vi "PointsToTiming.vi"(6 "Timing":T1 {"Pre-trigger length" format="%#_4p"; "Record length" format="%#_6p"; "Data rate" format="%#_6p"}, 7 "Device":T2, 8 "Pre-trigger position, %":dbl=1000000.0, 9 "Pre-trigger points":i64, 10 "Total points":i64, 11 "Actual Rate, Hz":dbl) -> (0 "Timing out":T1 {"Pre-trigger length" format="%#_4p"; "Record length" format="%#_6p"; "Data rate" format="%#_6p"}, 1 "Pre-trigger length, s":dbl, 2 "Record length, s":dbl, 3 "Data rate, Hz":dbl)   [LabVIEW 2015]
uses:
  Utilities/Controls/Timing Element.ctl
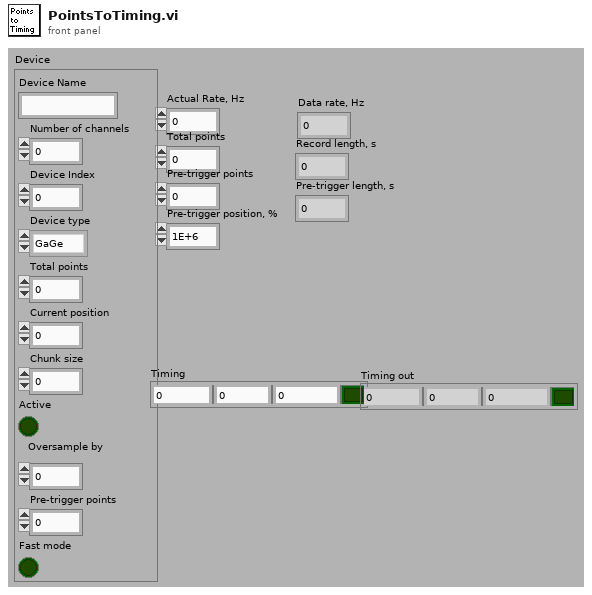
[diagram p1: front panel]
types:
  T1 = typedef "Timing Element.ctl" = cluster{"Data rate":dbl, "Record length":dbl, "Pre-trigger length":dbl, "Ext. clock":bool}
  T2 = cluster{"Device Name":string, "Number of channels":i32, "Device Index":i32, "Device type":enum16{"GaGe", "NI-DAQ", "NI-Scope", "CAMAC", "VXI-1433", "VXI-1437"}, "Total points":i64, "Current position":i64, "Chunk size":i64, "Active":bool, "Oversample by":i32, "Pre-trigger points":i64, "Fast mode":bool}
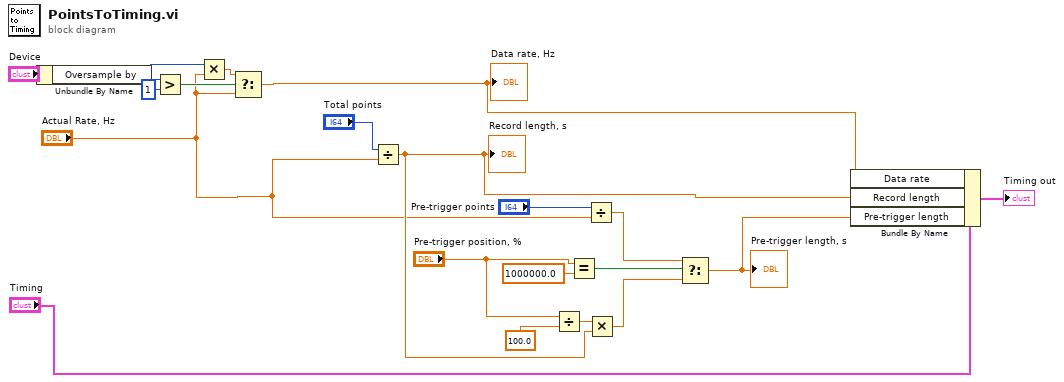
[diagram p0: block diagram]
diagram:
  n1 = Unbundle By Name("Device") -> ("Oversample by"=w2:i32)
  n2 = Greater?(x=w2, y=1) -> (0:w9:bool)
  n3 = Multiply(x=w2, y="Actual Rate, Hz") -> (x*y=w8:dbl)
  n4 = Select(t=w8, s=w9, f="Actual Rate, Hz") -> (s? t:f=w3:dbl)
  "Data rate, Hz" <- w3
  n5 = Divide(x="Total points", y="Actual Rate, Hz") -> (x/y=w4:dbl)
  "Record length, s" <- w4
  n6 = Divide(x="Pre-trigger position, %", y=100.0) -> (x/y=w20:dbl)
  n7 = Equal?(x="Pre-trigger position, %", y=1000000.0) -> (x = y?=w16:bool)
  n8 = Divide(x="Pre-trigger points", y="Actual Rate, Hz") -> (x/y=w15:dbl)
  n9 = Multiply(x=w20, y=w4) -> (x*y=w12:dbl)
  n10 = Select(t=w15, s=w16, f=w12) -> (s? t:f=w5:dbl)
  "Pre-trigger length, s" <- w5
  n11 = Bundle By Name(cluster="Timing", "Data rate"=w3, "Record length"=w4, "Pre-trigger length"=w5) -> (→"Timing out":T1)
